vi "Server1.vi"() -> ()   [LabVIEW 2020]
panel:
  in  "stop":bool
  # "VI Server"
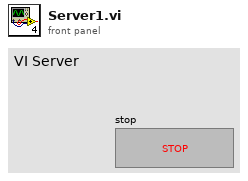
[diagram p1: front panel]
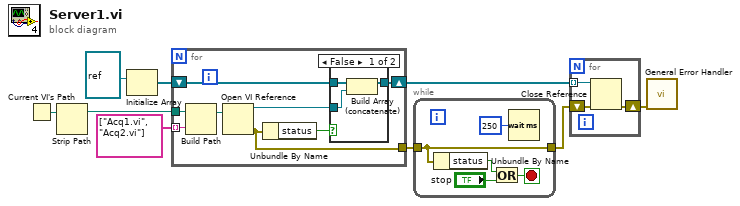
[diagram p0: block diagram]
diagram:
  n1 = Current VI's Path() -> (path=w5:path)
  n2 = Strip Path(path=w5) -> (stripped path=w4:path)  [unwired: 1 out]
  n3 = Initialize Array(refnum<vi> refnum) -> (w9:refnum<vi>[])  [unwired: 1 in]
  n4 = for {
    tunnel: string[] ["Acq1.vi", "Acq2.vi"] ("Server:VI Access List") -> [w16] mode=indexing
    shift-right: [w12] -> w6
    shift-left: w9 -> [w13]
    tunnel: w4 -> [w11]
    tunnel: [w10] -> w1
    n5 = Build Path(base path=w11, name or relative path=w16) -> (appended path=w17:path)
    n6 = Open VI Reference(vi path=w17) -> (vi reference=w14:refnum<vi>, error out=w10:errorcluster)  [unwired: 5 in]
    n7 = Unbundle By Name(w10) -> ("status"=w15:bool)
    n8 = case shown="False" w15 {
      tunnel: w14 -> [w18 _]
      tunnel: w13 -> [w20 w21]
      tunnel: [w19 w21] -> w12
      frame False {
        n9 = Build Array (concatenate)(w20, w18) -> (w19:refnum<vi>[])
      }
      frame True {
      }
    }
  }
  n10 = while {
    tunnel: w1 -> [w23]
    tunnel: [w23] -> w2
    stop <- w25 stop-if-true
    n11 = Unbundle By Name(w23) -> ("status"=w22:bool)
    n12 = Or(x=w22, y="stop") -> (x .or. y?=w25:bool)
    n13 = Wait (ms)(milliseconds to wait=u32 250) -> ()  [unwired: 1 out]
  }
  n14 = for {
    shift-right: [w28] -> w7
    shift-left: w2 -> [w29]
    tunnel: w6 -> [w27] mode=indexing
    n15 = Close Reference(reference=w27, error in (no error)=w29) -> (error out=w28:errorcluster)
  }
  n16 = call <vilib>:"General Error Handler.vi"("error in (no error)"=w7) -> ()  [unwired: 10 in, 5 out]
